vi "LWXPS_PositionerCompensationNotchModeFiltersSet.vi"(0 "Resonance frequency 1":dbl, 1 "Anti-resonance frequency 1":dbl, 2 "Resonance damping factor 1":dbl, 3 "Anti-resonance damping factor 1":dbl, 4 "Resonance frequency 2":dbl, 5 "Anti-resonance frequency 2":dbl, 6 "Positioner Name":string, 7 "Resonance damping factor 2":dbl, 8 "XPS Reference IN":refnum<k24>, 9 "Anti-resonance damping factor 2":dbl, 11 "LabVIEW error IN":errorcluster) -> (14 "XPS Reference OUT":refnum<k24>, 15 "Returned error code":i32, 18 "XPS Error String":string, 19 "LabVIEW error OUT":errorcluster)   [LabVIEW 2014]
uses:
  D:/XPSQ8_LabView_Library/Development/Source/Dll/Newport.XPS.CommandInterface.dll
  Dll/Newport.XPS.CommandInterface.dll
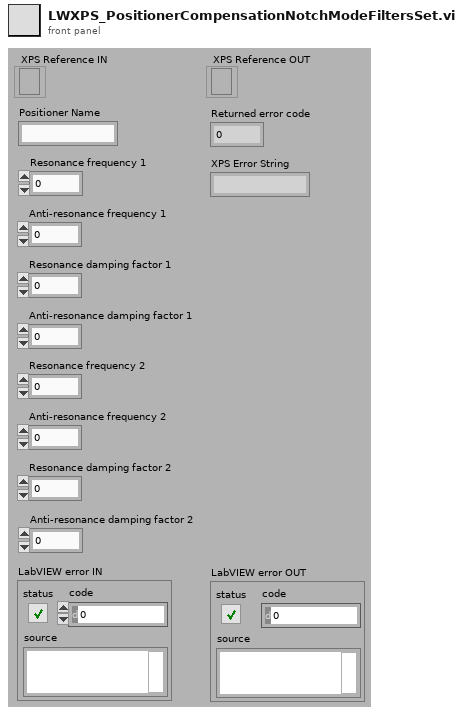
[diagram p1: front panel]
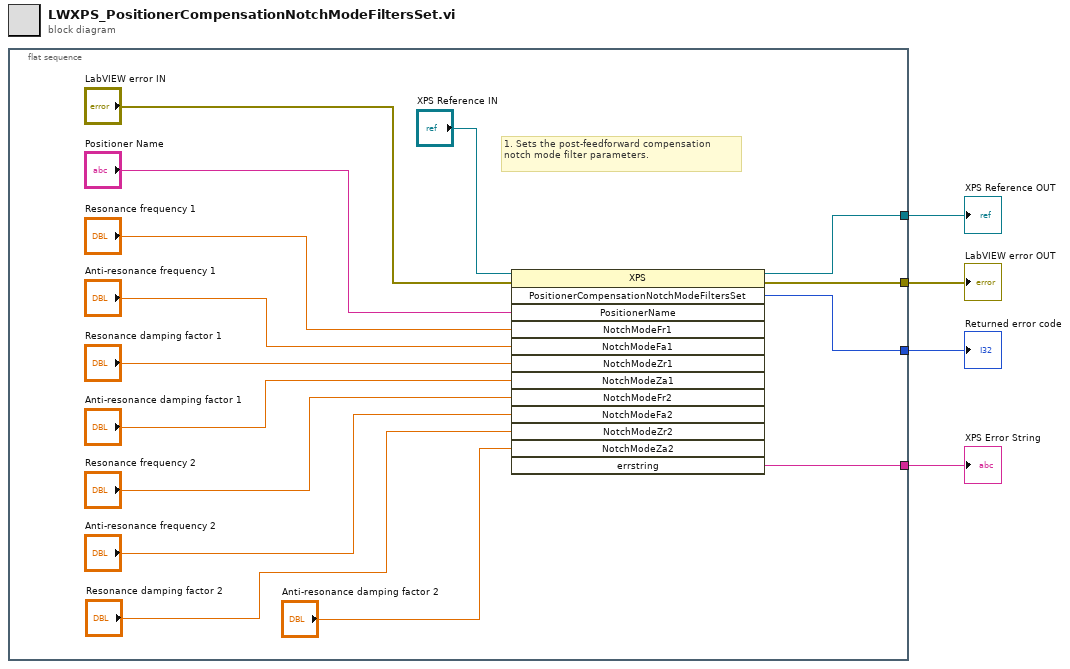
[diagram p0: block diagram]
diagram:
  n1 = flat-sequence {
    tunnel: [w16] -> w4
    tunnel: [w15] -> w3
    tunnel: [w17] -> w2
    tunnel: [w9] -> w1
    frame #0 {
      # "1. Sets the post-feedforward compensation notch mode filter parameters."
      n2 = invoke class="XPS" method="PositionerCompensationNotchModeFiltersSet"(reference="XPS Reference IN", error in="LabVIEW error IN", "PositionerName"="Positioner Name", "NotchModeFr1"="Resonance frequency 1", "NotchModeFa1"="Anti-resonance frequency 1", "NotchModeZr1"="Resonance damping factor 1", "NotchModeZa1"="Anti-resonance damping factor 1", "NotchModeFr2"="Resonance frequency 2", "NotchModeFa2"="Anti-resonance frequency 2", "NotchModeZr2"="Resonance damping factor 2", "NotchModeZa2"="Anti-resonance damping factor 2") -> (reference out=w16:refnum<k24>, error out=w15:errorcluster, "PositionerCompensationNotchModeFiltersSet"=w17:i32, "errstring"=w9:string)  [unwired: 2 in, 9 out]
    }
  }
  "XPS Error String" <- w1
  "XPS Reference OUT" <- w4
  "LabVIEW error OUT" <- w3
  "Returned error code" <- w2
